vi "Find Arduino.vi"(8 "error in (no error)":errorcluster) -> (0 "error out":errorcluster, 2 "Arduino Found?":bool, 3 "VISA resource name":refnum<visa-resource-name>)   [LabVIEW 2019, in "SHARED VI'S.lvlib"]
uses:
  <vilib>/Instr/_visa.llb/VISA Find Search Mode.ctl
  SHARED VI'S.lvlib
panel:
  out "match substring":string
  out "Array":string[](array[string])
  out "find list":string[](array[string])
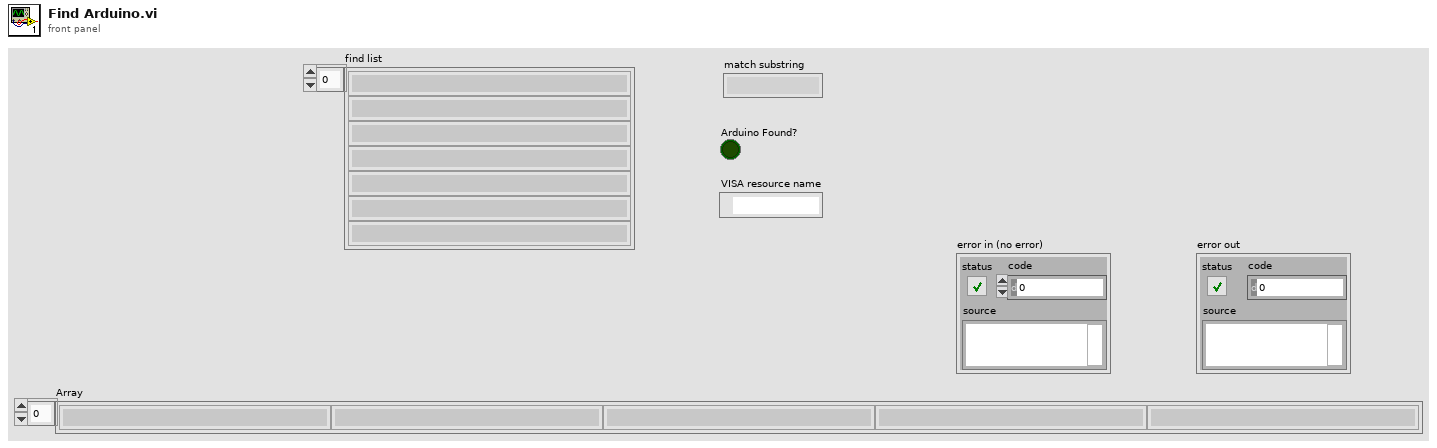
[diagram p1: front panel]
types:
  T1 = typedef "VISA Find Search Mode.ctl" = u32
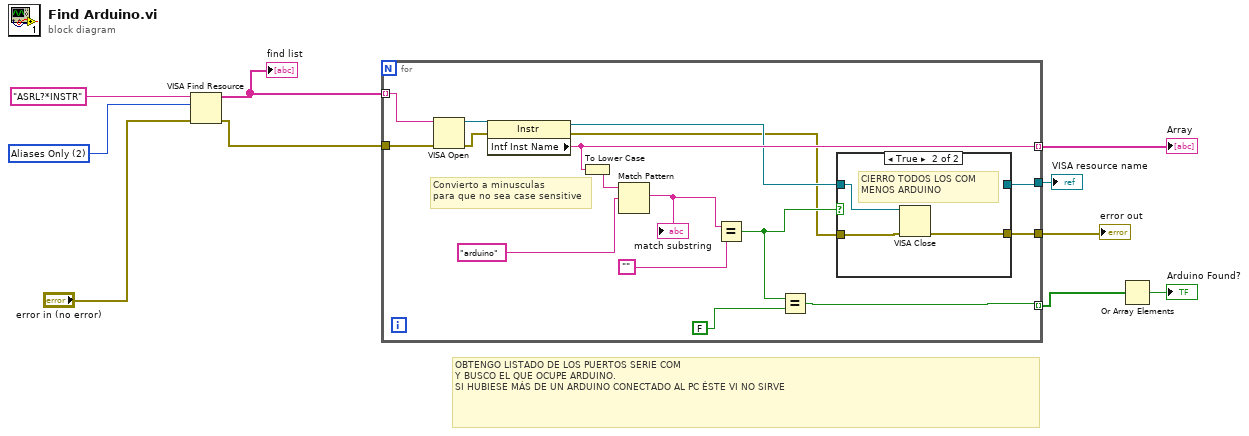
[diagram p0: block diagram]
diagram:
  w10 = T1 2 items=["Canonical Names Only"=0, "Aliases Only"=2, "Include Matching Aliases"=3, "Include All Aliases"=4] ("Search Mode")
  # "OBTENGO LISTADO DE LOS PUERTOS SERIE COM \nY BUSCO EL QUE OCUPE ARDUINO.\nSI HUBIESE MÁS DE UN ARDUINO CONECTADO AL PC ÉSTE VI NO SIRVE"
  n1 = VISA Find Resource(8:"error in (no error)", 10:w10, 11:"ASRL?*INSTR" ("expression (\"?*\")")) -> (0:w2:errorcluster, 3:w8:string[])  [unwired: 1 out]
  "find list" <- w8
  n2 = for {
    tunnel: w8 -> [w18] mode=indexing
    tunnel: [w22] -> w7 mode=indexing
    tunnel: [w15] -> w6 mode=indexing
    tunnel: [w13] -> w3
    tunnel: [w12] -> w4
    tunnel: w2 -> [w11]
    # "Convierto a minusculas\npara que no sea case sensitive"
    n3 = VISA Open(error in (no error)=w11, VISA resource name=w18) -> (VISA resource name=w26:refnum<visa-resource-name>, error out=w25:errorcluster)  [unwired: 3 in]
    n4 = property class="Instr"(reference=w26, error in=w25) -> (reference out=w19:refnum<visa-resource-name>, error out=w14:errorcluster, "Intf Inst Name"=w22:string)
    n5 = To Lower Case(string=w22) -> (all lower case string=w23:string)
    n6 = Match Pattern(string=w23, regular expression="arduino") -> (match substring=w21:string)  [unwired: 1 in, 3 out]
    "match substring" <- w21
    n7 = Equal?(x=w21, y="") -> (x = y?=w16:bool)
    n8 = Equal?(x=w16, y=FALSE) -> (x = y?=w15:bool)
    n9 = case shown="True" w16 {
      tunnel: w19 -> [w27 w31]
      tunnel: w14 -> [w28 w30]
      tunnel: [w28 w29] -> w13
      tunnel: [w27 _] -> w12
      frame False {
      }
      frame True {
        # "CIERRO TODOS LOS COM\nMENOS ARDUINO"
        n10 = VISA Close(VISA resource name=w31, error in (no error)=w30) -> (error out=w29:errorcluster)
      }
    }
  }
  "Array" <- w7
  "error out" <- w3
  "VISA resource name" <- w4
  n11 = Or Array Elements(Boolean array=w6) -> (logical OR=→"Arduino Found?":bool)
